vi "StreamInitPC.vi"() -> (0 "data cluster":T1={"Commands"=enum."Initialize", "Variant"=variant(enum16{"-90°", "+90°"} enum."-90°")}, 1 "reader name":string, 2 "writer name":string, 3 "writer buffer size":i32)   [LabVIEW 2017]
uses:
  TypeDefs/DataStreamCluster.ctl
  Projekt-RubikLibrary/CommandsRT.ctl
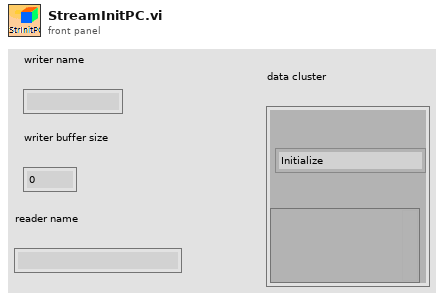
[diagram p1: front panel]
types:
  T1 = typedef "DataStreamCluster.ctl" = cluster{"Commands":T2, "Variant":variant}
  T2 = typedef "CommandsRT.ctl" = enum16{"Initialize", "Turn", "Grip", "Exit"}
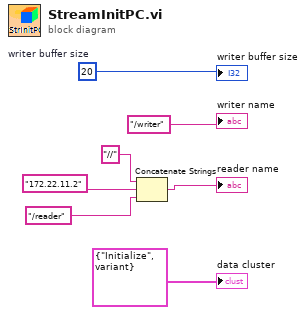
[diagram p0: block diagram]
diagram:
  w2 = 20  # writer buffer size
  n1 = Concatenate Strings("//", "172.22.11.2" ("myRIO IP Address"), "/reader") -> (→"reader name":string)
  "writer name" <- "/writer" ("reader name")
  "writer buffer size" <- w2
  "data cluster" <- T1 {"Commands"=enum."Initialize", "Variant"=variant(enum16{"-90°", "+90°"} enum."-90°")} ("data cluster")
